vi "Change Setting.vi"(8 "error in (no error)":errorcluster, 10 "Change setting mode":T1, 11 "Toggle 6 in":refnum<class "Toggle 7.1.lvclass">) -> (0 "error out":errorcluster, 1 "Changes":cluster{"Name":string, "Value":string}[](array[cluster]), 2 "Last setting":bool, 3 "Toggle 6 out":refnum<class "Toggle 7.1.lvclass">)   [LabVIEW 2020, in "Toggle 7.1.lvclass"]
uses:
  Toggle 7.1.lvclass
  Controls/Change setting mode enum.ctl
  PIC-device/PIC-Device.lvclass
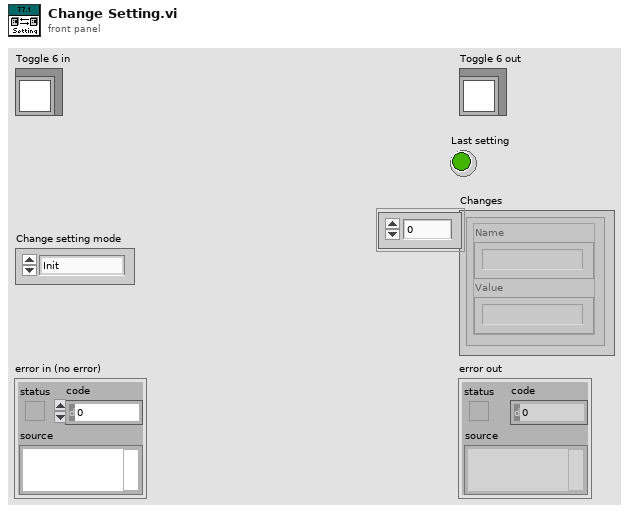
[diagram p1: front panel]
types:
  T1 = typedef "PIC-Device.lvclass/Change setting mode enum.ctl" = enum16{"Init", "Next", "Reset"}
  T2 = typedef "Toggle 7.1.lvclass/Test Sequence.ctl" = cluster{"Charge Pump Settings":T3[], "Charge Pump Values":dbl[], "Efuse Register Array":T3[], "Efuse Array":T4[], "Cap Register Array":T3[], "Cap Value Array":cluster{"Register Number":u32, "Value":dbl}[], "DWA Settings":T3[], "DWA Values":dbl[]}
  T3 = typedef "PIC-Device.lvclass/Register to Write.ctl" = cluster{"Register":u32, "Value":u32, "Dev Address":u32, "Physical Adress":u32}
  T4 = typedef "Toggle 7.1.lvclass/EFuse modes enum.ctl" = enum16{"On", "Off", "Both On and Off"}
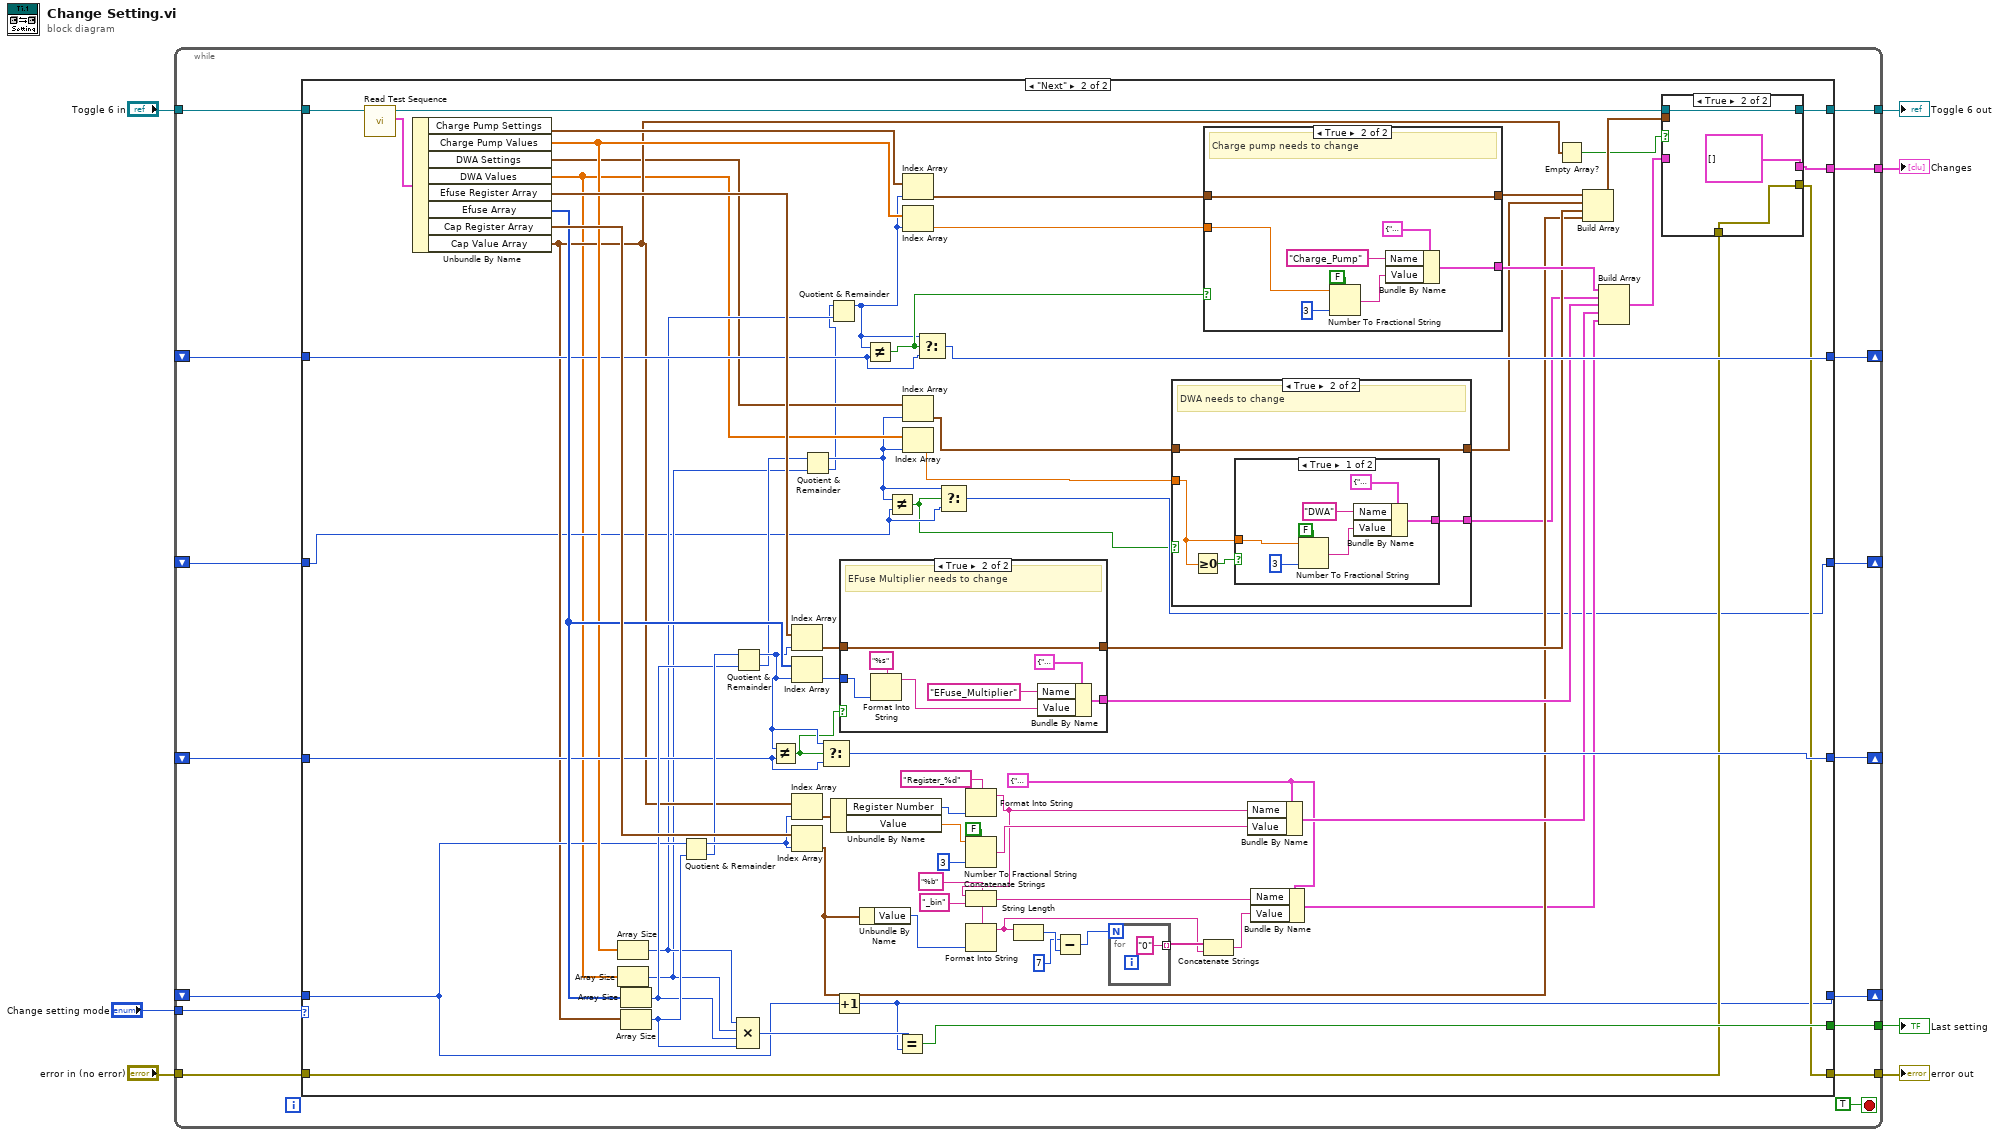
[diagram p0: block diagram]
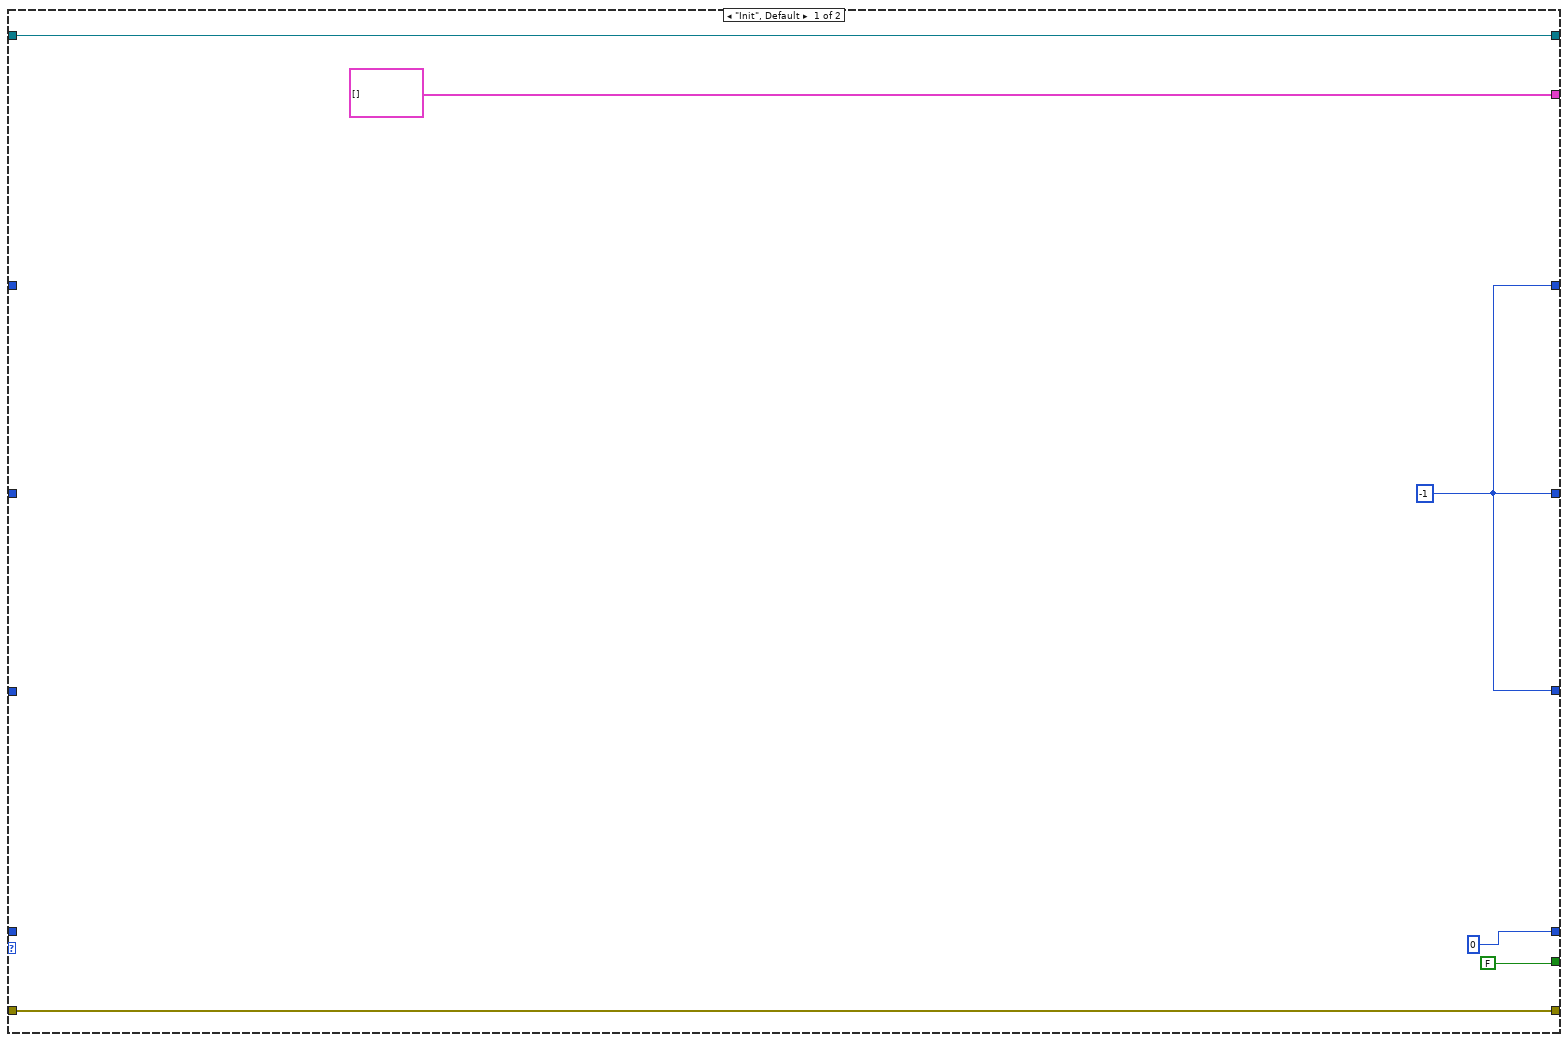
[diagram p2: hidden frame]
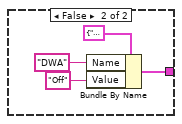
[diagram p4: hidden frame]
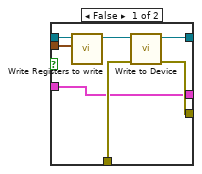
[diagram p5: hidden frame]
diagram:
  n1 = while {
    tunnel: "error in (no error)" -> [w21]
    tunnel: "Change setting mode" -> [w22]
    tunnel: "Toggle 6 in" -> [w17]
    tunnel: [w20] -> w4
    shift-right: [w19] -> _
    shift-left: _ -> [w18]
    tunnel: [w16] -> w3
    tunnel: [w15] -> w2
    shift-right: [w14] -> _
    shift-left: _ -> [w12]
    shift-right: [w13] -> _
    shift-left: _ -> [w11]
    tunnel: [w10] -> w1
    shift-right: [w9] -> _
    shift-left: _ -> [w8]
    stop <- TRUE stop-if-true
    n2 = case shown="\"Next\"" w22 {
      tunnel: w21 -> [w25 w67]
      tunnel: [FALSE w102] -> w20
      tunnel: [0 w44] -> w19
      tunnel: w18 -> [_ w49]
      tunnel: w17 -> [w26 w105]
      tunnel: [cluster{"Name":string, "Value":string}[] [] ("Changes") w46] -> w16
      tunnel: [w26 w68] -> w15
      tunnel: [w24 w86] -> w14
      tunnel: [w24 w79] -> w13
      tunnel: w12 -> [_ w87]
      tunnel: w11 -> [_ w80]
      tunnel: [w25 w66] -> w10
      tunnel: [w24 w39] -> w9
      tunnel: w8 -> [_ w40]
      frame "Init", Default {
        w24 = -1
      }
      frame "Next" {
        w62 = cluster{"Name":string, "Value":string} {"Name"="", "Value"=""} ("Change")
        n3 = call-dynamic "Read Test Sequence.vi"("Toggle 6 in"=w105) -> ("Test Sequence"=w104:T2, "Toggle 6 out"=w72:refnum<class "Toggle 7.1.lvclass">)  [unwired: 9 in]
        n4 = Unbundle By Name(w104) -> ("Charge Pump Settings"=w82:T3[], "Charge Pump Values"=w81:dbl[], "DWA Settings"=w37:T3[], "DWA Values"=w36:dbl[], "Efuse Register Array"=w90:T3[], "Efuse Array"=w89:T4[], "Cap Register Array"=w100:T3[], "Cap Value Array"=w48:cluster{"Register Number":u32, "Value":dbl}[])
        n5 = Array Size(array=w81) -> (size(s)=w43:i32)
        n6 = Array Size(array=w36) -> (size(s)=w41:i32)
        n7 = Array Size(array=w89) -> (size(s)=w91:i32)
        n8 = Array Size(array=w48) -> (size(s)=w101:i32)
        n9 = Quotient & Remainder(x=w49, y=w101) -> (x-y*floor(x/y)=w99:i32, floor(x/y)=w92:i32)
        n10 = Quotient & Remainder(x=w92, y=w91) -> (x-y*floor(x/y)=w88:i32, floor(x/y)=w42:i32)
        n11 = Compound Arithmetic op=MULTIPLY(w43, w41, w91, w101) -> (w103:i32)
        n12 = Not Equal?(x=w88, y=w87) -> (x != y?=w85:bool)
        n13 = Index Array(array=w90, index=w88) -> (element=w84:T3)
        n14 = Index Array(array=w89, index=w88) -> (element=w83:T4)
        n15 = Index Array(array=w48, index=w99) -> (element=w98:cluster{"Register Number":u32, "Value":dbl})
        n16 = Index Array(array=w100, index=w99) -> (element=w61:T3)
        n17 = Quotient & Remainder(x=w42, y=w41) -> (x-y*floor(x/y)=w35:i32, floor(x/y)=w34:i32)
        n18 = Select(t=w88, s=w85, f=w87) -> (s? t:f=w86:i32)
        n19 = Quotient & Remainder(x=w34, y=w43) -> (x-y*floor(x/y)=w65:i32)  [unwired: 1 out]
        n20 = Unbundle By Name(w98) -> ("Register Number"=w97:u32, "Value"=w94:dbl)
        n21 = Increment(x=w49) -> (x+1=w44:i32)
        n22 = case shown="True" w85 {
          tunnel: w84 -> [_ w140]
          tunnel: w83 -> [_ w145]
          tunnel: [_ w141] -> w74
          tunnel: [_ w140] -> w70
          frame False {
          }
          frame True {
            # "EFuse Multiplier needs to change"
            n23 = Format Into String(format string="%s", w145) -> (resulting string=w142:string)  [unwired: 2 in, 1 out]
            n24 = Bundle By Name(cluster=cluster{"Name":string, "Value":string} {"Name"="", "Value"=""} ("Change"), "Name"="EFuse_Multiplier", "Value"=w142) -> (w141:cluster{"Name":string, "Value":string})
          }
        }
        n25 = Unbundle By Name(w61) -> ("Value"=w59:u32)
        n26 = Not Equal?(x=w65, y=w80) -> (x != y?=w78:bool)
        n27 = Not Equal?(x=w35, y=w40) -> (x != y?=w38:bool)
        n28 = Equal?(x=w103, y=w44) -> (x = y?=w102:bool)
        n29 = Index Array(array=w82, index=w65) -> (element=w77:T3)
        n30 = Index Array(array=w81, index=w65) -> (element=w76:dbl)
        n31 = Index Array(array=w37, index=w35) -> (element=w33:T3)
        n32 = Index Array(array=w36, index=w35) -> (element=w32:dbl)
        n33 = Select(t=w65, s=w78, f=w80) -> (s? t:f=w79:i32)
        n34 = Select(t=w35, s=w38, f=w40) -> (s? t:f=w39:i32)
        n35 = Format Into String(format string="Register_%d", w97) -> (resulting string=w64:string)  [unwired: 2 in, 1 out]
        n36 = Number To Fractional String(use system decimal point (T)=FALSE, number=w94, precision (6)=i16 3) -> (F-format string=w95:string)  [unwired: 1 in]
        n37 = Concatenate Strings(w64, "_bin" ("string")) -> (w60:string)
        n38 = Format Into String(format string="%b", w59) -> (resulting string=w52:string)  [unwired: 2 in, 1 out]
        n39 = String Length(string=w52) -> (length=w56:i32)
        n40 = Subtract(x=7, y=w56) -> (x-y=w54:i32)
        n41 = for {
          N: w54 -> [_]
          tunnel: ["0"] -> w53 mode=indexing
        }
        n42 = case shown="True" w38 {
          tunnel: w33 -> [_ w109]
          tunnel: w32 -> [_ w106]
          tunnel: [_ w109] -> w30
          tunnel: [_ w108] -> w31
          frame False {
          }
          frame True {
            # "DWA needs to change"
            n43 = Greater Or Equal To 0?(x=w106) -> (x >= 0?=w107:bool)
            n44 = case shown="True" w107 {
              tunnel: [w112 w118] -> w108
              tunnel: w106 -> [w110 _]
              frame True {
                n45 = Number To Fractional String(use system decimal point (T)=FALSE, number=w110, precision (6)=i16 3) -> (F-format string=w114:string)  [unwired: 1 in]
                n46 = Bundle By Name(cluster=cluster{"Name":string, "Value":string} {"Name"="", "Value"=""} ("Change"), "Name"="DWA", "Value"=w114) -> (w112:cluster{"Name":string, "Value":string})
              }
              frame False {
                n47 = Bundle By Name(cluster=cluster{"Name":string, "Value":string} {"Name"="", "Value"=""} ("Change"), "Name"="DWA", "Value"="Off") -> (w118:cluster{"Name":string, "Value":string})
              }
            }
          }
        }
        n48 = case shown="True" w78 {
          tunnel: w77 -> [_ w134]
          tunnel: w76 -> [_ w135]
          tunnel: [_ w134] -> w71
          tunnel: [_ w133] -> w75
          frame False {
          }
          frame True {
            # "Charge pump needs to change"
            n49 = Number To Fractional String(use system decimal point (T)=FALSE, number=w135, precision (6)=i16 3) -> (F-format string=w137:string)  [unwired: 1 in]
            n50 = Bundle By Name(cluster=cluster{"Name":string, "Value":string} {"Name"="", "Value"=""} ("Change"), "Name"="Charge_Pump", "Value"=w137) -> (w133:cluster{"Name":string, "Value":string})
          }
        }
        n51 = Concatenate Strings(w53, w52) -> (w51:string)
        n52 = Bundle By Name(cluster=w62, "Name"=w64, "Value"=w95) -> (w73:cluster{"Name":string, "Value":string})
        n53 = Bundle By Name(cluster=w62, "Name"=w60, "Value"=w51) -> (w57:cluster{"Name":string, "Value":string})
        n54 = Empty Array?(array=w48) -> (empty?=w47:bool)
        n55 = Build Array(w71, w30, w70, w61) -> (w69:T3[])
        n56 = Build Array(w75, w31, w74, w73, w57) -> (w45:cluster{"Name":string, "Value":string}[])
        n57 = case shown="True" w47 {
          tunnel: w72 -> [w127 w130]
          tunnel: w69 -> [w126 _]
          tunnel: [w124 w130] -> w68
          tunnel: w67 -> [w123 w129]
          tunnel: [w122 w129] -> w66
          tunnel: [w121 cluster{"Name":string, "Value":string}[] []] -> w46
          tunnel: w45 -> [w121 _]
          frame False {
            n58 = call-dynamic "Write Registers to write.vi"("Registers to write"=w126, "Device in"=w127) -> ("Device out"=w125:refnum<class "Toggle 7.1.lvclass">)  [unwired: 9 in]
            n59 = call-dynamic "Write to Device.vi"("error in (no error)"=w123, "Device in"=w125) -> ("error out"=w122:errorcluster, "Device out"=w124:refnum<class "Toggle 7.1.lvclass">)  [unwired: 7 in, 1 out]
          }
          frame True {
          }
        }
      }
    }
  }
  "error out" <- w1
  "Toggle 6 out" <- w2
  "Changes" <- w3
  "Last setting" <- w4
